vi "190625_Simulation_FreCTO.vi"() -> ()   [LabVIEW 2015]
uses:
  <vilib>/Utility/Variable/NI_VariableUtilities.lvlib
panel:
  in  "X_Type":string(combo)="Notch15"
  in  "X_pole":string(combo)="4352"
  in  "Z_Type":string(combo)="Notch15"
  in  "Z_pole":string(combo)="4952"
  out "all time(s)":dbl
  out "Time slots (sec)":dbl[](array[numeric]) format="%#.10f"
  in  "Sample Rate (Hz)":dbl=1000.0 format="%#_13g"
  in  "STOP":bool
  in  "Load":bool
  in  "CLEAR":bool
  in  "RUN":bool
  out "RMS  X (um)":dbl format="%0.2f"
  out "MAX  X (um)":dbl format="%0.2f"
  out "RMS (one) X (um)":dbl format="%0.2f"
  out "Output X (mm)":dbl[](graph)
  out "CMD X (mm)":dbl[](graph)
  out "Position Error X (um)":dbl[](graph)
  out "Position Command X (mm)":dbl[](graph)
  out "time length":i32=15000
  out "start time":i32=7500
  out "RMS (one) Z (um)":dbl format="%0.2f"
  out "MAX  Z (um)":dbl format="%0.2f"
  out "RMS  Z (um)":dbl format="%0.2f"
  out "Position Error Z (um)":dbl[](graph)
  out "CMD Z (mm)":dbl[](graph)
  out "Output Z (mm)":dbl[](graph)
  out "Position Command Z (mm)":dbl[](graph)
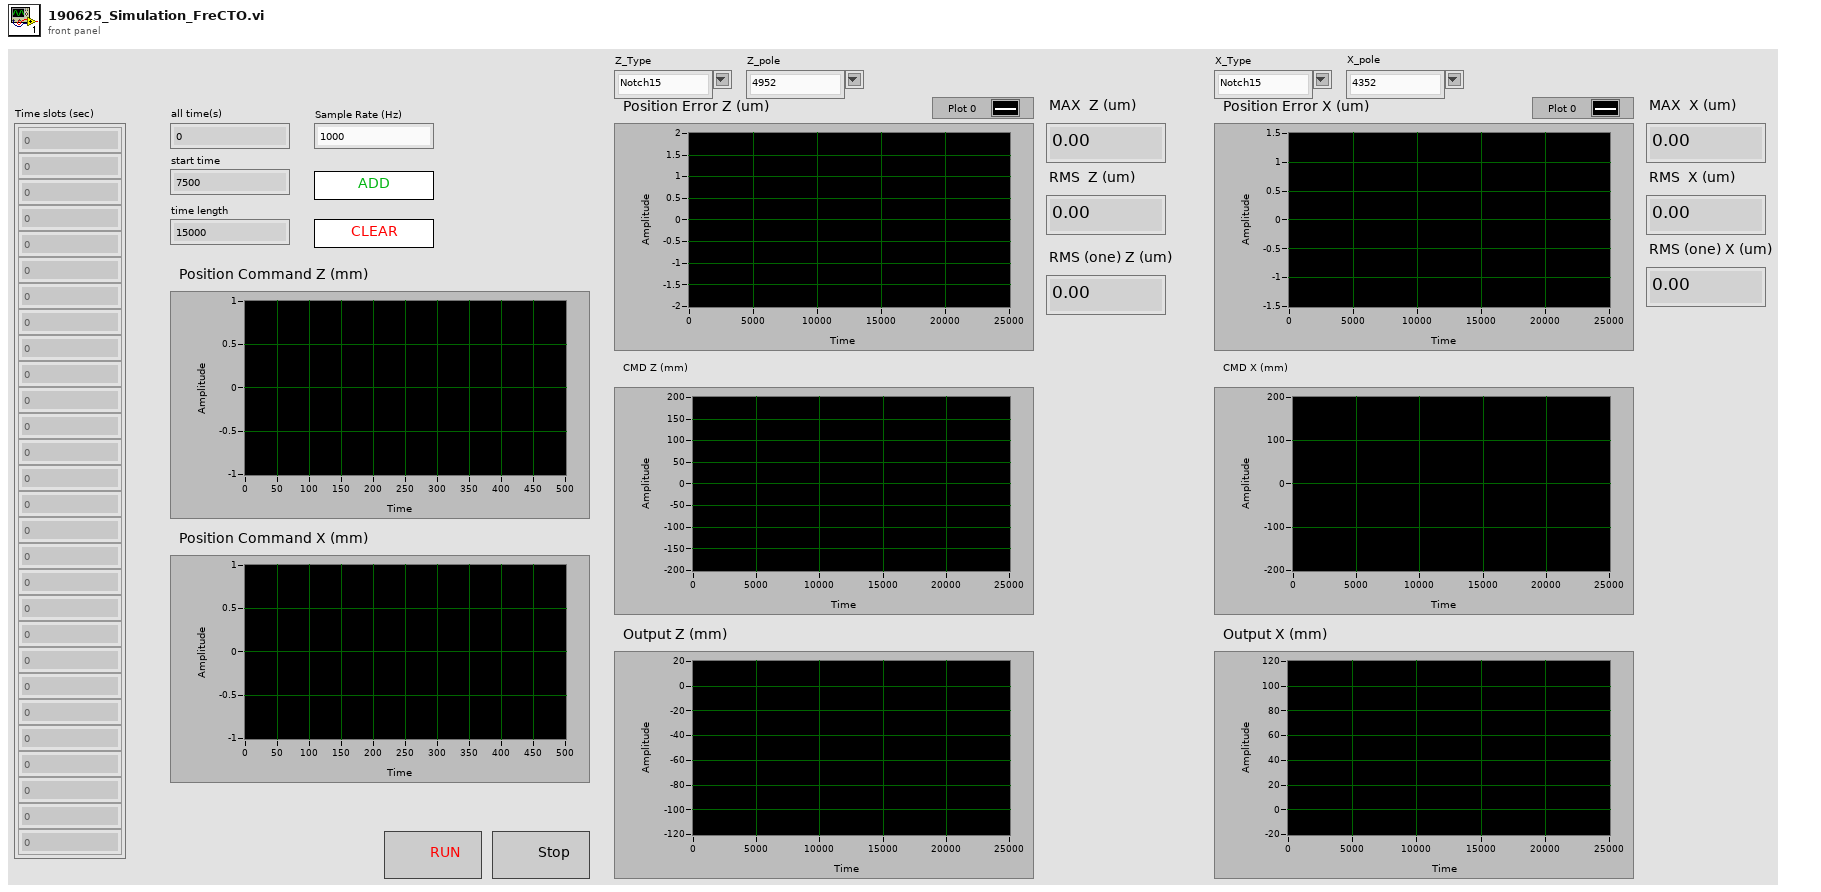
[diagram p1: front panel]
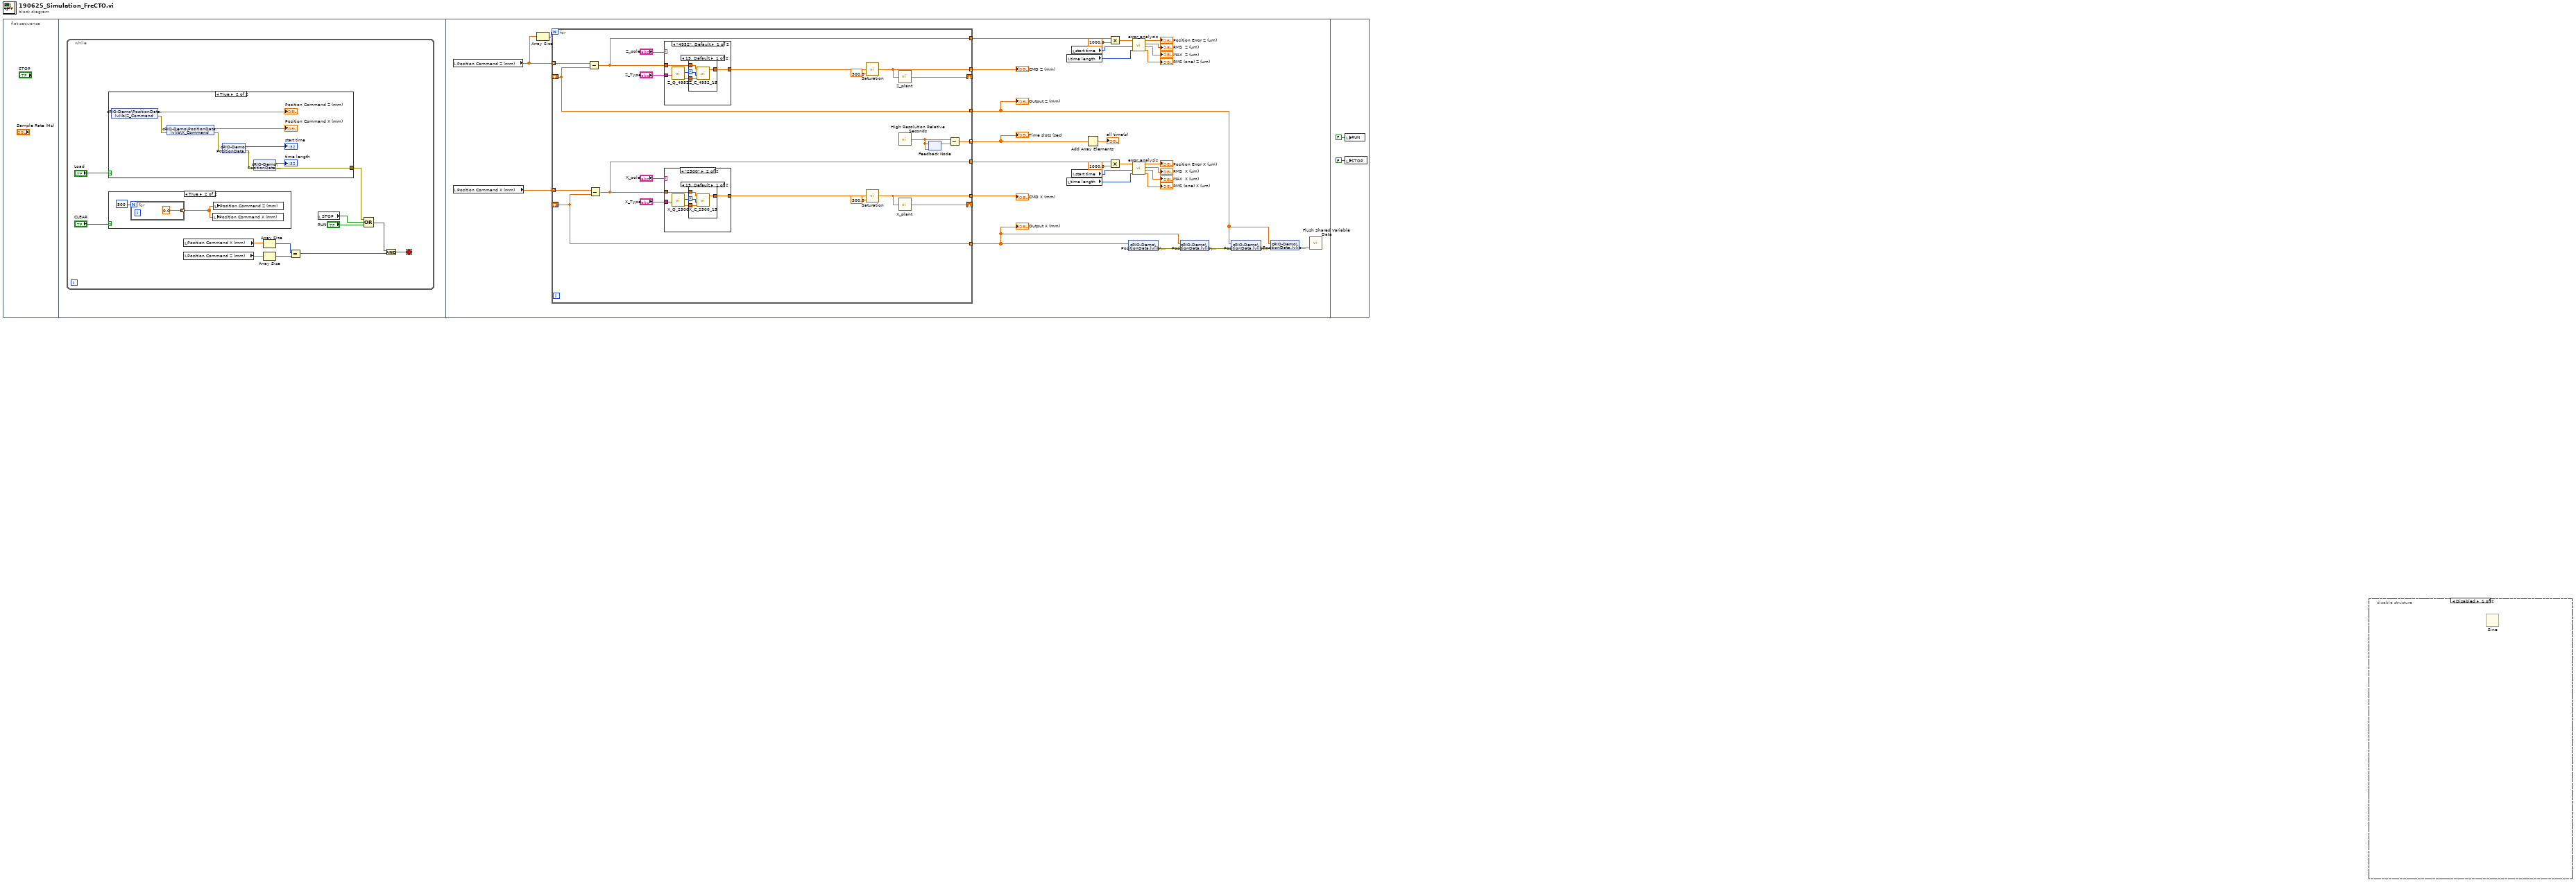
[diagram p0: block diagram]
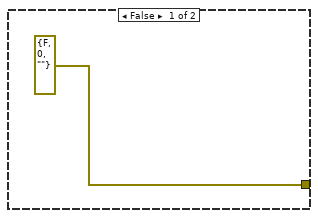
[diagram p3: hidden frame]
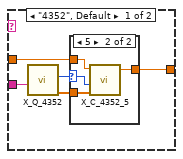
[diagram p4: hidden frame]
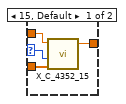
[diagram p5: hidden frame]
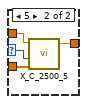
[diagram p6: hidden frame]
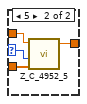
[diagram p7: hidden frame]
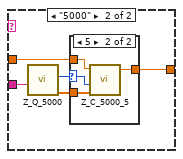
[diagram p8: hidden frame]
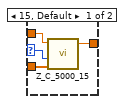
[diagram p9: hidden frame]
diagram:
  n1 = flat-sequence {
    frame #0 {
    }
    frame #1 {
      n2 = while {
        stop <- w9 stop-if-true
        n3 = case shown="True" "Load" {
          tunnel: [errorcluster {"status"=FALSE, "code"=0, "source"=""} ("error IO") w19] -> w1
          frame False {
          }
          frame True {
            n4 = shared-variable "cRIO-Demo\\PositionData.lvlib\\Z_Command"() -> (→"Position Command Z (mm)":dbl[], error out=w22:errorcluster)  [unwired: 1 in]
            n5 = shared-variable "cRIO-Demo\\PositionData.lvlib\\X_Command"(error in=w22) -> (→"Position Command X (mm)":dbl[], error out=w20:errorcluster)
            n6 = shared-variable "cRIO-Demo\\PositionData.lvlib\\t0"(error in=w20) -> (→"start time":i32, error out=w21:errorcluster)
            n7 = shared-variable "cRIO-Demo\\PositionData.lvlib\\tL"(error in=w21) -> (→"time length":i32, error out=w19:errorcluster)
          }
        }
        n8 = case shown="True" "CLEAR" {
          frame False {
          }
          frame True {
            n9 = for {
              N: 500 -> [_]
              tunnel: [0.0 ("element")] -> w14 mode=indexing
            }
            n10 = local write "Position Command X (mm)"(w14) -> ()
            n11 = local write "Position Command Z (mm)"(w14) -> ()
          }
        }
        n12 = local read "Position Command X (mm)"() -> (w10:dbl[])
        n13 = local read "Position Command Z (mm)"() -> (w11:dbl[])
        n14 = Array Size(array=w11) -> (size(s)=w7:i32)
        n15 = Array Size(array=w10) -> (size(s)=w8:i32)
        n16 = Equal?(x=w8, y=w7) -> (x = y?=w6:bool)
        n17 = local read "STOP"() -> (w2:bool)
        n18 = Compound Arithmetic op=OR(w1, w2, "RUN") -> (w4:bool)
        n19 = And(x=w4, y=w6) -> (x .and. y?=w9:bool)
      }
    }
    frame #2 {
      n20 = local read "Position Command Z (mm)"() -> (w54:dbl[])
      n21 = local read "Position Command X (mm)"() -> (w38:dbl[])
      n22 = Array Size(array=w54) -> (size(s)=w53:i32)
      n23 = for {
        N: w53 -> [_]
        shift-right: [w70] -> _
        shift-left: _ -> [w65]
        tunnel: [w65] -> w26 mode=indexing
        tunnel: [w62] -> w34 mode=indexing
        tunnel: [w69] -> w55 mode=indexing
        tunnel: w54 -> [w67] mode=indexing
        tunnel: w38 -> [w66] mode=indexing
        shift-right: [w71] -> _
        shift-left: _ -> [w57]
        tunnel: [w72] -> w37 mode=indexing
        tunnel: [w59] -> w32 mode=indexing
        tunnel: [w57] -> w27 mode=indexing
        tunnel: [w73] -> w36 mode=indexing
        n24 = Subtract(x=w67, y=w65) -> (x-y=w62:dbl)
        n25 = Subtract(x=w66, y=w57) -> (x-y=w59:dbl)
        n26 = case shown="\"4952\", Default" "Z_pole" {
          tunnel: "Z_Type" -> [w107 w120]
          tunnel: w62 -> [w104 w117]
          tunnel: [w103 w116] -> w61
          frame "4952", Default {
            n27 = call "Z_Q_4952.vi"("Type"=w107) -> ("Qn"=w105:dbl[], "L"=w106:i32)  [unwired: 9 in]
            n28 = case shown="15, Default" w106 {
              selector: w106 -> [w109 w113]
              tunnel: w105 -> [w108 w112]
              tunnel: w104 -> [w111 w115]
              tunnel: [w110 w114] -> w103
              frame 15, Default {
                n29 = call "Z_C_4952_15.vi"("ek"=w111, "length"=w109, "q"=w108) -> ("uk"=w110:dbl)  [unwired: 4 in]
              }
              frame 5 {
                n30 = call "Z_C_4952_5.vi"("ek"=w115, "length"=w113, "q"=w112) -> ("uk"=w114:dbl)  [unwired: 4 in]
              }
            }
          }
          frame "5000" {
            n31 = call "Z_Q_5000.vi"("Type"=w120) -> ("Qn"=w118:dbl[], "L"=w119:i32)  [unwired: 9 in]
            n32 = case shown="5" w119 {
              selector: w119 -> [w122 w126]
              tunnel: w118 -> [w121 w125]
              tunnel: w117 -> [w124 w128]
              tunnel: [w123 w127] -> w116
              frame 15, Default {
                n33 = call "Z_C_5000_15.vi"("ek"=w124, "length"=w122, "q"=w121) -> ("uk"=w123:dbl)  [unwired: 4 in]
              }
              frame 5 {
                n34 = call "Z_C_5000_5.vi"("ek"=w128, "length"=w126, "q"=w125) -> ("uk"=w127:dbl)  [unwired: 4 in]
              }
            }
          }
        }
        n35 = case shown="\"2500\"" "X_pole" {
          tunnel: "X_Type" -> [w81 w94]
          tunnel: w59 -> [w78 w91]
          tunnel: [w77 w90] -> w58
          frame "4352", Default {
            n36 = call "X_Q_4352.vi"("Type"=w81) -> ("Qn"=w79:dbl[], "L"=w80:i32)  [unwired: 9 in]
            n37 = case shown="5" w80 {
              selector: w80 -> [w83 w87]
              tunnel: w79 -> [w82 w86]
              tunnel: w78 -> [w85 w89]
              tunnel: [w84 w88] -> w77
              frame 15, Default {
                n38 = call "X_C_4352_15.vi"("ek"=w85, "length"=w83, "q"=w82) -> ("uk"=w84:dbl)  [unwired: 4 in]
              }
              frame 5 {
                n39 = call "X_C_4352_5.vi"("ek"=w89, "length"=w87, "q"=w86) -> ("uk"=w88:dbl)  [unwired: 4 in]
              }
            }
          }
          frame "2500" {
            n40 = call "X_Q_2500.vi"("Type"=w94) -> ("Qn"=w92:dbl[], "L"=w93:i32)  [unwired: 9 in]
            n41 = case shown="15, Default" w93 {
              selector: w93 -> [w96 w100]
              tunnel: w92 -> [w95 w99]
              tunnel: w91 -> [w98 w102]
              tunnel: [w97 w101] -> w90
              frame 15, Default {
                n42 = call "X_C_2500_15.vi"("ek"=w98, "length"=w96, "q"=w95) -> ("uk"=w97:dbl)  [unwired: 4 in]
              }
              frame 5 {
                n43 = call "X_C_2500_5.vi"("ek"=w102, "length"=w100, "q"=w99) -> ("uk"=w101:dbl)  [unwired: 4 in]
              }
            }
          }
        }
        n44 = call "Saturation.vi"("Vmax"=300.0, "uk"=w61) -> ("real uk"=w69:dbl)  [unwired: 3 in]
        n45 = call "Saturation.vi"("Vmax"=300.0, "uk"=w58) -> ("real uk"=w72:dbl)  [unwired: 3 in]
        n46 = call "Z_plant.vi"("u"=w69) -> ("y"=w70:dbl)  [unwired: 4 in]
        n47 = call <vilib>:"High Resolution Relative Seconds.vi"() -> ("relative seconds"=w68:dbl)
        n48 = call "X_plant.vi"("u"=w72) -> ("y"=w71:dbl)  [unwired: 4 in]
        n49 = feedback #1(w68) -> (w74:dbl)
        n50 = feedback-in #1(w68) -> ()
        n51 = Subtract(x=w68, y=w74) -> (x-y=w73:dbl)
      }
      "Output Z (mm)" <- w26
      "CMD Z (mm)" <- w55
      "Output X (mm)" <- w27
      "CMD X (mm)" <- w37
      "Time slots (sec)" <- w36
      n52 = local read "time length"() -> (w48:i32)
      n53 = local read "time length"() -> (w42:i32)
      n54 = local read "start time"() -> (w47:i32)
      n55 = local read "start time"() -> (w41:i32)
      n56 = Add Array Elements(numeric array=w36) -> (sum=→"all time(s)":dbl)
      n57 = Multiply(x=w34, y=1000.0) -> (x*y=w46:dbl[])
      n58 = Multiply(x=w32, y=1000.0) -> (x*y=w39:dbl[])
      n59 = shared-variable "cRIO-Demo\\PositionData.lvlib\\X_EN"(w27) -> (error out=w29:errorcluster)  [unwired: 1 in]
      n60 = call "error_analysis.vi"("tLength"=w48, "t0"=w47, "data in (um)"=w46) -> ("rms (one) (um)"=→"RMS (one) Z (um)":dbl, "max err (um)"=→"MAX  Z (um)":dbl, "rms (all) (um)"=→"RMS  Z (um)":dbl, "data out (um)"=→"Position Error Z (um)":dbl[])  [unwired: 5 in]
      n61 = call "error_analysis.vi"("tLength"=w42, "t0"=w41, "data in (um)"=w39) -> ("rms (one) (um)"=→"RMS (one) X (um)":dbl, "max err (um)"=→"MAX  X (um)":dbl, "rms (all) (um)"=→"RMS  X (um)":dbl, "data out (um)"=→"Position Error X (um)":dbl[])  [unwired: 5 in]
      n62 = shared-variable "cRIO-Demo\\PositionData.lvlib\\X_LS"(w27, error in=w29) -> (error out=w28:errorcluster)
      n63 = shared-variable "cRIO-Demo\\PositionData.lvlib\\Z_EN"(w26, error in=w28) -> (error out=w30:errorcluster)
      n64 = shared-variable "cRIO-Demo\\PositionData.lvlib\\Z_LS"(w26, error in=w30) -> (error out=w25:errorcluster)
      n65 = call <vilib>:"Flush Shared Variable Data.vi"("error in (no error)"=w25) -> ()  [unwired: 10 in, 1 out]
    }
    frame #3 {
      n66 = local write "RUN"(FALSE ("RUN")) -> ()
      n67 = local write "STOP"(FALSE ("STOP")) -> ()
    }
  }
  n68 = disable-structure shown="Disabled" {
    frame Disabled {
      n69 = Sine() -> ()  [unwired: 1 in, 1 out]
    }
    frame Enabled {
    }
  }
